vi "Write Device Command.vi"(8 "error in (no error)":errorcluster, 10 "Device Command":T1(ring), 11 "VISA resource name":refnum<visa-resource-name>) -> (0 "error out":errorcluster, 3 "VISA resource name out":refnum<visa-resource-name>)   [LabVIEW 2012, in "Temptronic TP04300.lvlib"]
doc: "This VI writes a device specific command to the TP04300 instrument.\n\nThe following commands are supported:\n\n<b>TP04300_AIR_FLOW</b> - turns the main air flow On or Off, depending on the Command Argument value.\n Use Command Argument \n = 0 to turn the air flow off\n = 1 to turn the air flow on\n\n[TP04300_TRICKLE_FLOW] - turns the trickle air flow On or Off, depending on the Command Argument value.\n\n Use Command Argument \n = 0 to turn the trickle flow off\n = 1 to turn the trickle flow on\n \n[TP04300_HEAD] - moves the head Up or Down, depending on the Command Argument value.\n\n Use Command Argument \n = 0 to move the head Up\n = 1 to move the head Down\n\n[TP04300_HEAD_LOCK] - allows to lock/unlock the head position, depending on the Command Argument value.\n\n Use Command Argument \n = 0 to unlock the head\n = 1 to lock the head\n\n[TP04300_COMPRESSOR] - turns the compressor On or Off, depending on the Command Argument value.\n\n Use Command Argument \n = 0 to turn the compressor off\n = 1 to turn the compressor on"
uses:
  <instrlib>/Temptronic TP04300/Temptronic TP04300.lvlib
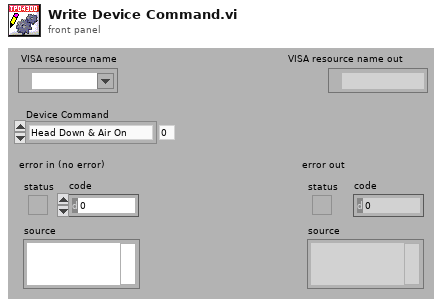
[diagram p1: front panel]
types:
  T1 = enum16{"Head Down & Air On", "Head Up & Air Off", "Air Flow Off", "Air Flow On", "Trickle Flow Off", "Trickle Flow On", "Head Up", "Head Down", "Head Lock Off", "Head Lock On", "Compressor Off", "Compressor On"}
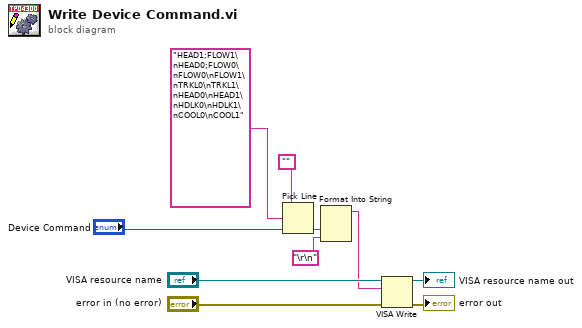
[diagram p0: block diagram]
diagram:
  n1 = Pick Line(string ("")="", multi-line string="HEAD1;FLOW1\nHEAD0;FLOW0\nFLOW0\nFLOW1\nTRKL0\nTRKL1\nHEAD0\nHEAD1\nHDLK0\nHDLK1\nCOOL0\nCOOL1", line index="Device Command") -> (output string=w4:string)
  n2 = Format Into String(w4, "\r\n") -> (resulting string=w2:string)  [unwired: 3 in, 1 out]
  n3 = VISA Write(VISA resource name="VISA resource name", write buffer=w2, error in (no error)="error in (no error)") -> (VISA resource name out=→"VISA resource name out":refnum<visa-resource-name>, error out=→"error out":errorcluster)  [unwired: 1 out]
